vi "SetOutput.vi"(3 "State":bool, 4 "error in":errorcluster, 5 "connection ID":refnum<k5>) -> (1 "error out":errorcluster, 2 "connection ID out":refnum<k5>)   [LabVIEW 2013]
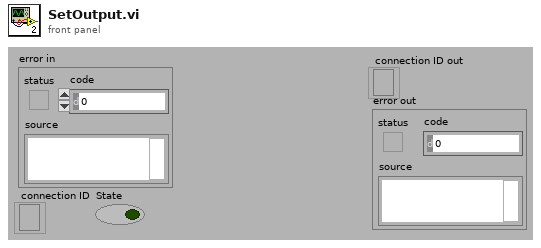
[diagram p1: front panel]
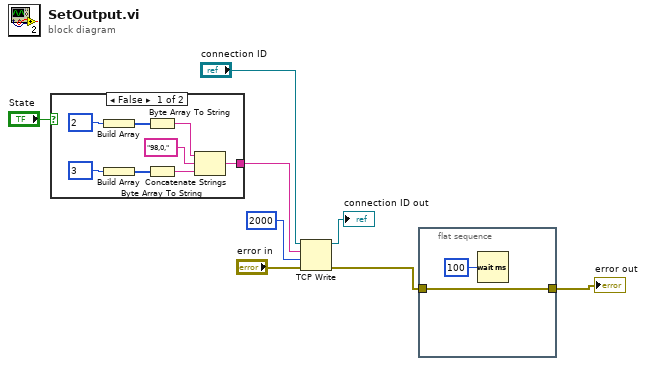
[diagram p0: block diagram]
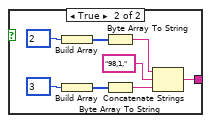
[diagram p2: hidden frame]
diagram:
  n1 = case shown="False" "State" {
    tunnel: [w9 w17] -> w3
    frame False {
      n2 = Build Array(u8 2 ("y")) -> (w15:u8[])
      n3 = Build Array(u8 3 ("y")) -> (w11:u8[])
      n4 = Byte Array To String(unsigned byte array=w15) -> (string=w14:string)
      n5 = Byte Array To String(unsigned byte array=w11) -> (string=w10:string)
      n6 = Concatenate Strings(w14, "98,0," ("string"), w10) -> (w9:string)
    }
    frame True {
      n7 = Build Array(u8 2 ("y")) -> (w23:u8[])
      n8 = Build Array(u8 3 ("y")) -> (w19:u8[])
      n9 = Byte Array To String(unsigned byte array=w23) -> (string=w22:string)
      n10 = Byte Array To String(unsigned byte array=w19) -> (string=w18:string)
      n11 = Concatenate Strings(w22, "98,1," ("string"), w18) -> (w17:string)
    }
  }
  n12 = TCP Write(connection ID="connection ID", data in=w3, error in (no error)="error in", 9:2000 ("timeout ms (25000)")) -> (connection ID out=→"connection ID out":refnum<k5>, error out=w2:errorcluster)  [unwired: 1 out]
  n13 = flat-sequence {
    tunnel: [w26] -> w1
    tunnel: w2 -> [w26]
    frame #0 {
      n14 = Wait (ms)(milliseconds to wait=u32 100) -> ()  [unwired: 1 out]
    }
  }
  "error out" <- w1
